vi "Configure Frequency (Center Span).vi"(0 "VISA resource name":refnum<visa-resource-name>, 5 "Center Frequency (3000000000Hz)":dbl=3000000000.0 min=-100000000.0 max=43100000000.0, 7 "Span Frequency (25000000Hz)":dbl=25000000.0 min=0.0 max=43200000000.0, 11 "error in (no error)":errorcluster) -> (4 "VISA resource name out":refnum<visa-resource-name>, 15 "error out":errorcluster)   [LabVIEW 2023, in "Anritsu Signal Analyzer Series.lvlib"]
doc: "Configures the frequency range of the spectrum analyzer using the center frequency and the frequency span\n\n<B>Note:</B>\nThis command is not available during the Spurious Emission (Mask) measurement or the Spurious Emission measurement."
uses:
  Anritsu Signal Analyzer Series.lvlib
panel:
  out "resulting string":string
  # "Hz"
  # "Hz"
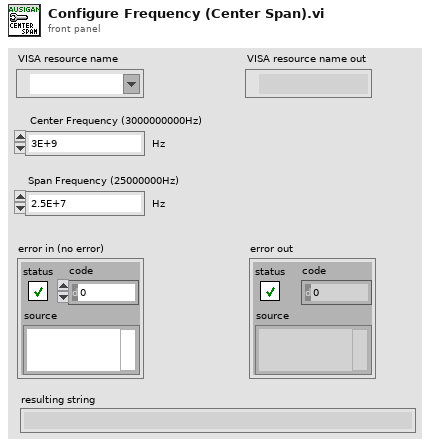
[diagram p1: front panel]
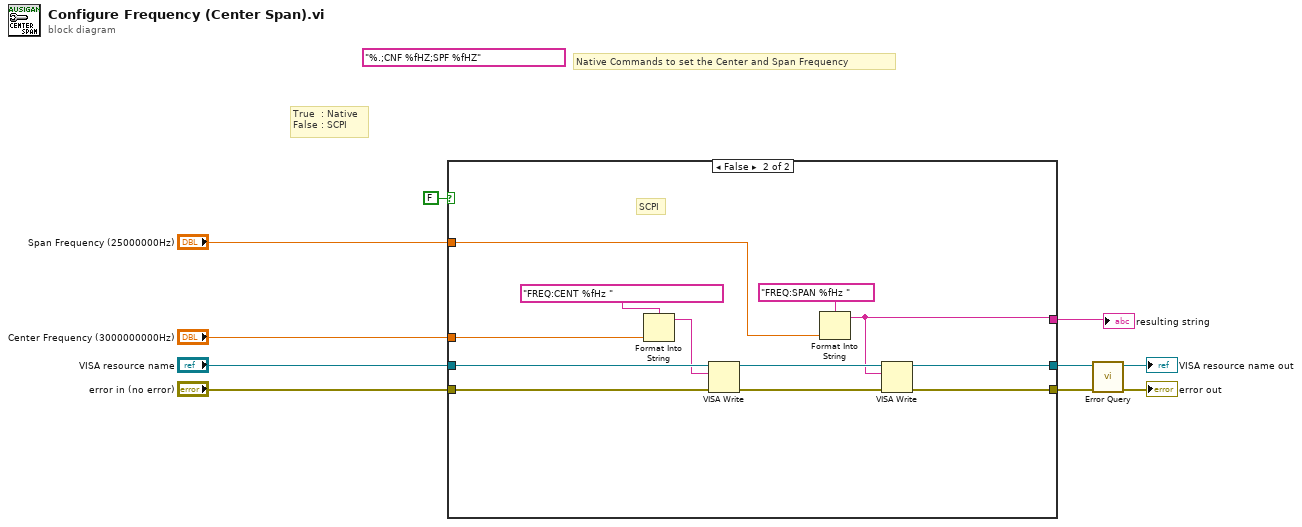
[diagram p0: block diagram]
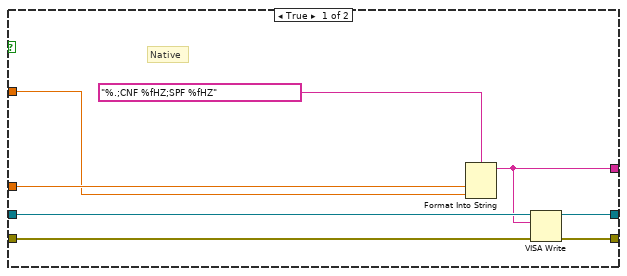
[diagram p2: hidden frame]
diagram:
  (unwired) "%.;CNF %fHZ;SPF %fHZ" ("Format String")
  # "True  : Native\nFalse : SCPI"
  # "Native Commands to set the Center and Span Frequency"
  n1 = case shown="False" FALSE {
    tunnel: "Center Frequency (3000000000Hz)" -> [w18 w30]
    tunnel: "VISA resource name" -> [w17 w29]
    tunnel: "error in (no error)" -> [w16 w28]
    tunnel: [w14 w24] -> w5
    tunnel: "Span Frequency (25000000Hz)" -> [w12 w22]
    tunnel: [w15 w20] -> w3
    tunnel: [w11 w19] -> w1
    frame True {
      # "Native"
      n2 = Format Into String(format string="%.;CNF %fHZ;SPF %fHZ" ("Format String"), w18, w12) -> (resulting string=w11:string)  [unwired: 2 in, 1 out]
      n3 = VISA Write(VISA resource name=w17, write buffer=w11, error in (no error)=w16) -> (VISA resource name out=w15:refnum<visa-resource-name>, error out=w14:errorcluster)  [unwired: 1 out]
    }
    frame False {
      # "SCPI"
      n4 = Format Into String(format string="FREQ:CENT %fHz " ("Format String"), w30) -> (resulting string=w26:string)  [unwired: 2 in, 1 out]
      n5 = VISA Write(VISA resource name=w29, write buffer=w26, error in (no error)=w28) -> (VISA resource name out=w21:refnum<visa-resource-name>, error out=w25:errorcluster)  [unwired: 1 out]
      n6 = Format Into String(format string="FREQ:SPAN %fHz " ("Format String"), w22) -> (resulting string=w19:string)  [unwired: 2 in, 1 out]
      n7 = VISA Write(VISA resource name=w21, write buffer=w19, error in (no error)=w25) -> (VISA resource name out=w20:refnum<visa-resource-name>, error out=w24:errorcluster)  [unwired: 1 out]
    }
  }
  "resulting string" <- w1
  n8 = call "Error Query.vi"("error in (no error)"=w5, "VISA resource name"=w3) -> ("error out"=→"error out":errorcluster, "VISA resource name out"=→"VISA resource name out":refnum<visa-resource-name>)  [unwired: 6 in, 2 out]
